vi "Spectral Density.vi"() -> ()   [LabVIEW 2015]
uses:
  <vilib>/addons/_NISVFA/_Spectrum Processing/SVFA Spectrum Peak Search (1 Ch).vi
  <vilib>/addons/_NISVFA/_Spectrum Processing/subVIs/svfa_Spectrum Peak Search.vi
  <vilib>/addons/_NISVFA/_Shared subVIs/Common/svc_Spectrum Units.vi
  <vilib>/addons/_NISVFA/_Spectrum Processing/subVIs/svfa_Peak Rough Search Indices.vi
  <vilib>/addons/_NISVFA/_Subset FFT/SVFA Power Spectrum Subset (1 Ch).vi
  <vilib>/addons/_NISVFA/_Spectrum Processing/subVIs/svfa_Three Finger Peak Search.vi
  <vilib>/addons/_NISVFA/_Shared subVIs/Common/svc_Format Value (DBL).vi
  <vilib>/addons/_NISVFA/_Shared subVIs/Common/svc_Engineering Units to Unit Label.vi
  <vilib>/addons/_NISVFA/_Shared subVIs/Common/svc_Unit Label Lexical Class.vi
  <vilib>/addons/_NISVFA/_Shared subVIs/Common/svc_Get Weighting Enum and Labels.vi
  <vilib>/addons/_NISVFA/_Shared subVIs/Common/svc_Caller VI Returned in Error Source.vi
panel:
  in  "stop 2":bool
  out "Boolean 2":bool
  out "Boolean":bool
  out "Array 3":dbl[](array[numeric])
  out "Array 2":dbl[](array[numeric])
  out "Array":dbl[](array[numeric])
  out "number of peaks":i32
  in  "Peak search type":u16(ring)=1 items=["Peak Search 0", "Peak Search 1"]
  in  "PSD type":u16(ring) items=["PSD 0", "PSD 1"]
  in  "Threshold":dbl=-28.0
  in  "Min Scale":dbl
  in  "Max Scale":dbl=10000.0
  out "peaks":cluster{"freq. or order":dbl, "value":dbl}[](array[cluster])=[{"freq. or order"=99.99850804277241, "value"=-0.7926774419152083}, {"freq. or order"=1000.0, "value"=-20.789519028935615}, {"freq. or order"=2500.180930647048, "value"=-26.722435636658822}] {"value" format="%#.1g"; "freq. or order" format="%#_4g"}
  in  "stop":bool
  out "Waveform Graph":cluster{"x0":dbl, "dx":dbl, "magnitude":dbl[]}(graph)={"x0"=0.0, "dx"=10.0, "magnitude"=array[5000 elements]}
  # "Power Spectral Density"
  # "Threshold"
  # "Peaks"
  # "Magnitude"
  # "Frequency"
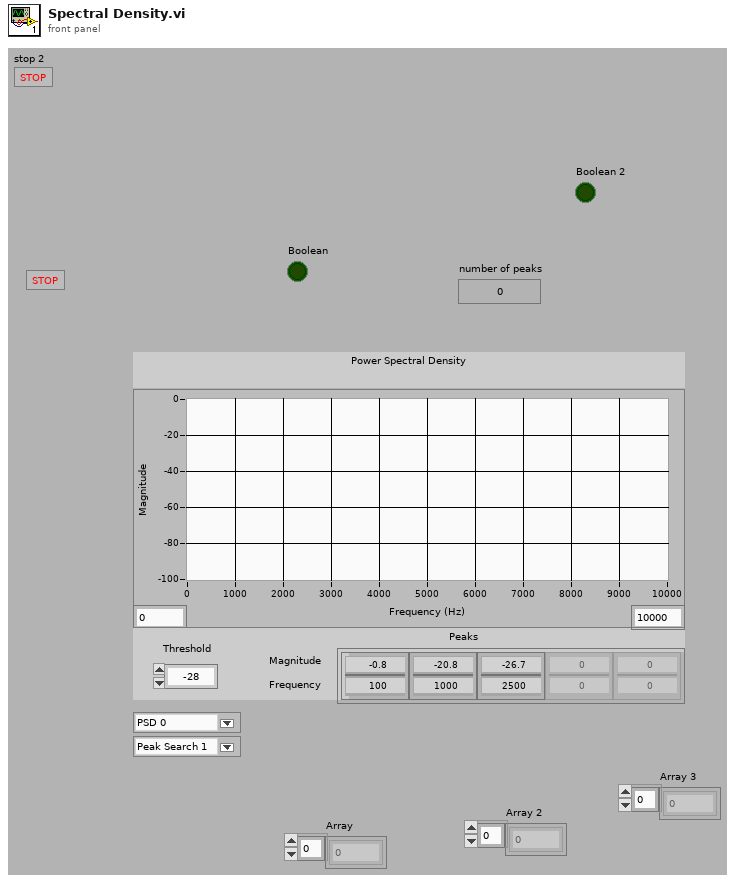
[diagram p1: front panel]
types:
  T1 = cluster{"single/multiple":enum16{"Multiple Peaks", "Single Max Peak"}, "Threshold":dbl}
  T2 = typedef "svc_Spectrum Info.ctl" = cluster{"channel name":string, "description":string, "x-axis units":T3, "spectral info":cluster{"spectrum type":T4, "linear/dB":enum16{"linear", "dB"}, "window":u16, "window size":i32, "FFT size":i32}, "engineering units":T5, "custom label":string, "dB reference [EU]":dbl, "peak units":enum16{"rms", "peak", "peak-peak"}, "weighting filter":T6, "spectral density?":bool, "unit label":string, "spectrum skewed?":bool, "complimentary spectrum units":T7}
  T3 = typedef "svc_X-Axis Units.ctl" = u16
  T4 = typedef "svc_Spectrum Type.ctl" = enum16{"FFT Spectrum [complex]", "Amplitude [Magnitude]", "Power [Magnitude^2]", "Cross Spectrum [complex]", "Frequency Response [Complex]"}
  T5 = typedef "svc_Engineering Units Text Ring.ctl" = u16
  T6 = typedef "svc_Weighting Filter Text Ring.ctl" = u16
  T7 = typedef "svc_Complimentary Spectrum Units.ctl" = enum16{"none", "radians", "degrees", "cycles", "imaginary"}
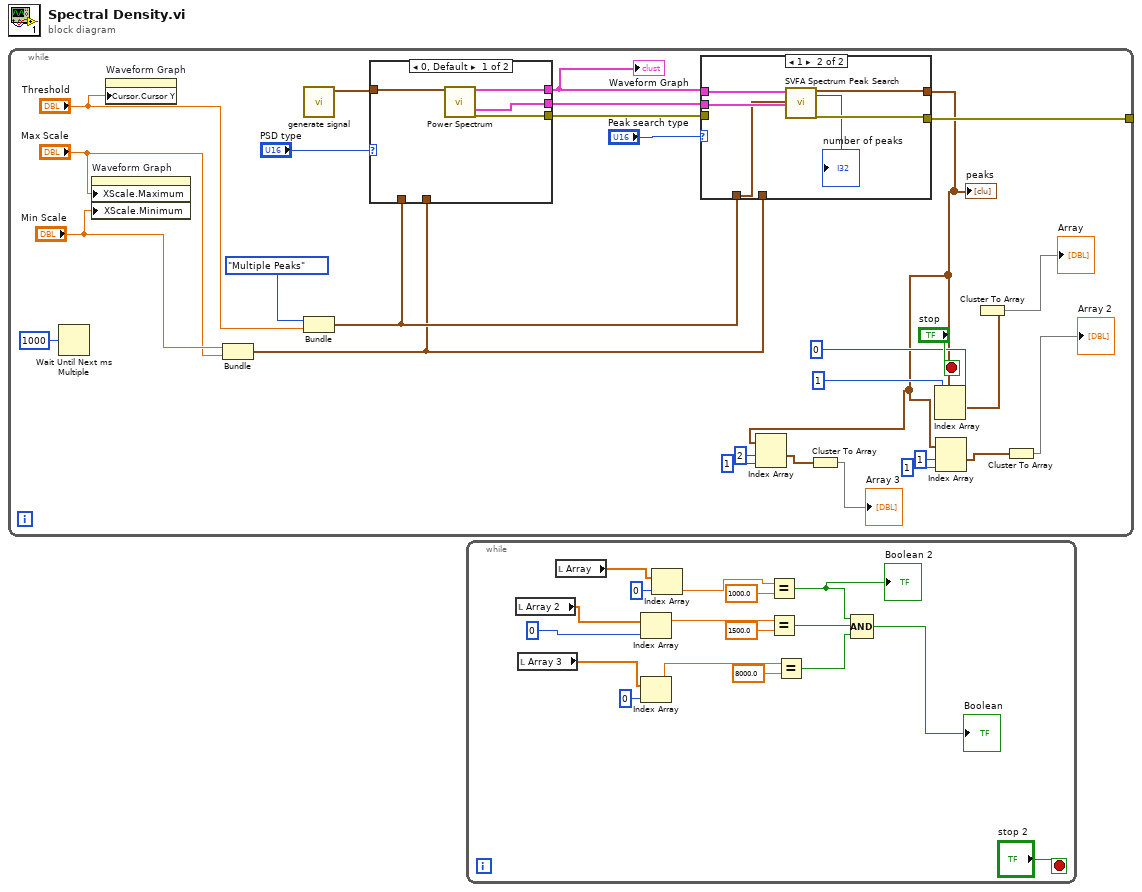
[diagram p0: block diagram]
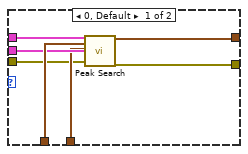
[diagram p2: hidden frame]
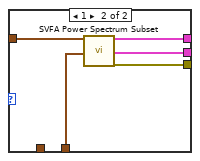
[diagram p3: hidden frame]
diagram:
  n1 = while {
    tunnel: [w14] -> _
    stop <- "stop" stop-if-true
    n2 = Wait Until Next ms Multiple(millisecond multiple=u32 1000) -> ()  [unwired: 1 out]
    n3 = property on="Waveform Graph" class="WFGraph (strict)"("XScale.Maximum"="Max Scale", "XScale.Minimum"="Min Scale") -> ()  [unwired: 2 in, 2 out]
    n4 = property on="Waveform Graph" class="WFGraph (strict)"("Cursor.Cursor Y"="Threshold") -> ()  [unwired: 2 in, 2 out]
    n5 = Bundle("Min Scale"="Min Scale", "Max Scale"="Max Scale") -> (w18:cluster{"Min Scale":dbl, "Max Scale":dbl})  [unwired: 1 in]
    n6 = call "generate signal.vi"() -> ("Waveform Graph 5"=w24:waveform(dbl))  [unwired: 11 in]
    n7 = Bundle("single/multiple"=enum16{"Multiple Peaks", "Single Max Peak"}."Multiple Peaks", "Threshold"="Threshold") -> (w19:T1)  [unwired: 1 in]
    n8 = case shown="0, Default" "PSD type" {
      tunnel: w24 -> [w45 w48]
      tunnel: [w44 w50] -> w22
      tunnel: [w43 w49] -> w23
      tunnel: w19 -> [_ _]
      tunnel: w18 -> [_ w47]
      tunnel: [w42 w46] -> w15
      frame 0, Default {
        n9 = call "Power Spectrum"("input signal"=w45) -> ("spectrum"=w44:cluster{"x0":dbl, "dx":dbl, "magnitude":dbl[]}, "spectrum info"=w43:T2, "error out"=w42:errorcluster)  [unwired: 13 in, 3 out]
      }
      frame 1 {
        n10 = call-poly <vilib>:"SVFA Power Spectrum Subset.vi"("scaled signal [EU]"=w48, "frequency range"=w47) -> ("power spectrum [dB EU]"=w50:cluster{"f0":dbl, "df":dbl, "magnitude":dbl[]}, "spectrum info"=w49:T2, "error out"=w46:errorcluster)  [unwired: 12 in, 3 out]
      }
    }
    "Waveform Graph" <- w22
    n11 = case shown="1" "Peak search type" {
      tunnel: w22 -> [w35 w41]
      tunnel: w19 -> [w34 w38]
      tunnel: w23 -> [w33 w40]
      tunnel: w18 -> [w32 _]
      tunnel: [w31 w39] -> w5
      tunnel: w15 -> [w30 _]
      tunnel: [w29 w37] -> w14
      frame 0, Default {
        n12 = call "Peak Search"("input spectrum"=w35, "peak search settings"=w34, "frequency range"=w32, "spectrum info"=w33, "error in"=w30) -> ("peaks"=w31:cluster{"freq. or order":dbl, "value":dbl}[], "error out"=w29:errorcluster)  [unwired: 11 in, 2 out]
      }
      frame 1 {
        n13 = call-poly <vilib>:"SVFA Spectrum Peak Search.vi"("spectrum"=w41, "peak search settings"=w38, "spectrum info in"=w40) -> ("peaks"=w39:cluster{"freq. or order":dbl, "value":dbl}[], "number of peaks"=→"number of peaks":i32, "error out"=w37:errorcluster)  [unwired: 12 in, 2 out]
      }
    }
    "peaks" <- w5
    n14 = Index Array(array=w5, index #1=2 ("index"), index #2=1 ("index")) -> (element #1=w2:cluster{"freq. or order":dbl, "value":dbl})  [unwired: 1 out]
    n15 = Cluster To Array(cluster=w2) -> (array=→"Array 3":dbl[])
    n16 = Index Array(array=w5, index #1=0 ("index"), index #2=1 ("index")) -> (element #1=w11:cluster{"freq. or order":dbl, "value":dbl})  [unwired: 1 out]
    n17 = Index Array(array=w5, index #1=1 ("index"), index #2=1 ("index")) -> (element #1=w7:cluster{"freq. or order":dbl, "value":dbl})  [unwired: 1 out]
    n18 = Cluster To Array(cluster=w11) -> (array=→"Array":dbl[])
    n19 = Cluster To Array(cluster=w7) -> (array=→"Array 2":dbl[])
  }
  n20 = while {
    stop <- "stop 2" stop-if-true
    n21 = local read "Array 2"() -> (w61:dbl[])
    n22 = local read "Array 3"() -> (w59:dbl[])
    n23 = local read "Array"() -> (w64:dbl[])
    n24 = Index Array(array=w61, index=0) -> (element=w60:dbl)
    n25 = Index Array(array=w59, index=0) -> (element=w57:dbl)
    n26 = Index Array(array=w64, index=0) -> (element=w63:dbl)
    n27 = Equal?(x=w63, y=1000.0) -> (x = y?=w52:bool)
    "Boolean 2" <- w52
    n28 = Equal?(x=w60, y=1500.0) -> (x = y?=w53:bool)
    n29 = Equal?(x=w57, y=8000.0) -> (x = y?=w66:bool)
    n30 = Compound Arithmetic op=AND(w52, w53, w66) -> (→"Boolean":bool)
  }
